vi "pumpsec_09_3.vi"(0 "reset":i32, 1 "master":i32, 2 "correction":dbl=1.0, 3 "manual":i32, 4 "pause":i32, 5 "Port":i32=10, 6 "pump_type":i32, 7 "port, Reglo D":i32, 10 "Target":dbl[](array[numeric])=[10.0, 2.0, 0.0, 0.0, 0.0, 0.0, 0.0, 0.0, 0.0, 0.0], 12 "fr_manual":dbl, 13 "Time":dbl[](array[numeric])=[4.0, 2.0, 0.0, 0.0, 0.0, 0.0, 0.0, 0.0, 0.0, 0.0]) -> (11 "Reglo D":dbl, 14 "Scale":dbl, 15 "mA":dbl format="%#_2g", 17 "Scale actual":dbl, 18 "params":dbl[](array[numeric]), 19 "PAM":dbl)   [LabVIEW 2015]
uses:
  BERTTA.dll
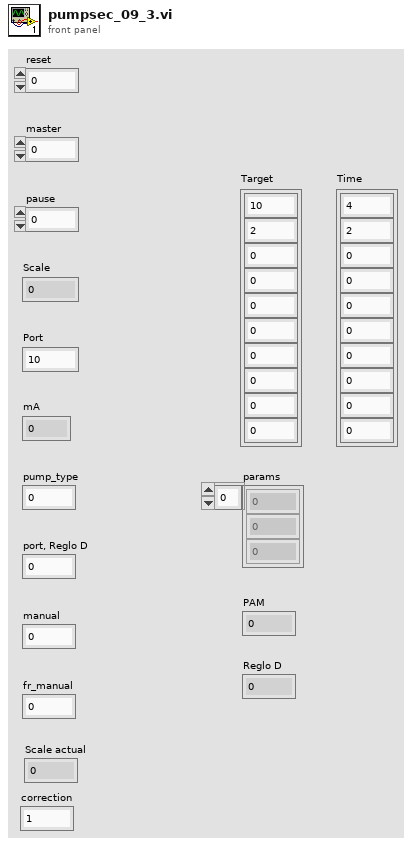
[diagram p1: front panel]
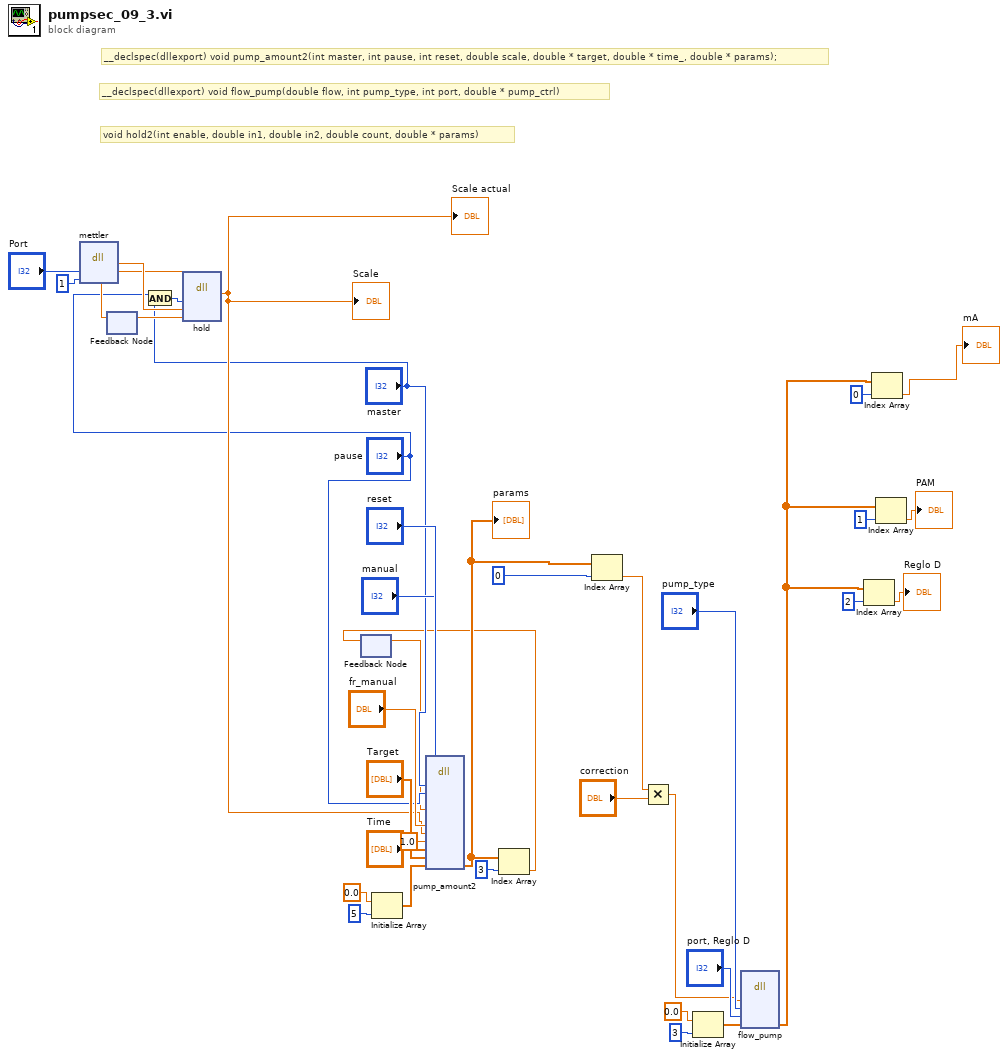
[diagram p0: block diagram]
diagram:
  # "void hold2(int enable, double in1, double in2, double count, double * params)"
  # "__declspec(dllexport) void flow_pump(double flow, int pump_type, int port, double * pump_ctrl)"
  # "__declspec(dllexport) void pump_amount2(int master, int pause, int reset, double scale, double * target, double * time_, double * params);"
  n1 = dll-call lib="C:/Users/shresplab/OneDrive - Kemira Oyj/Documents/Visual Studio 2017/Projects/Bertta/BERTTA/x64/Debug/BERTTA.dll" fn="mettler"("port"="Port", "msg"=1) -> ("return type"=w14:dbl)  [unwired: 5 in, 2 out]
  n2 = feedback #1() -> (w13:dbl)  [unwired: 1 in]
  n3 = And(x="pause", y="master") -> (x .and. y?=w9:i32)
  n4 = dll-call lib="C:/Users/shresplab/OneDrive - Kemira Oyj/Documents/Visual Studio 2017/Projects/Bertta/BERTTA/x64/Debug/BERTTA.dll" fn="hold"("enable"=w9, "in1"=w14, "in2"=w13) -> ("return type"=w12:dbl)  [unwired: 6 in, 2 out]
  "Scale" <- w12
  "Scale actual" <- w12
  n5 = feedback-in #1(w12) -> ()
  n6 = feedback #2() -> (w5:dbl)  [unwired: 1 in]
  n7 = Initialize Array(0.0 ("element"), 5 ("dimension size")) -> (w22:dbl[])
  n8 = dll-call lib="C:/Users/shresplab/OneDrive - Kemira Oyj/Documents/Visual Studio 2017/Projects/Bertta/BERTTA/x64/Debug/BERTTA.dll" fn="pump_amount2"("master"="master", "pause"="pause", "reset"="reset", "count"=w5, "manual"="manual", "fr_manual"="fr_manual", "scale"=w12, "elapsed"=1.0, "target"="Target", "time_"="Time", "params"=w22) -> ("params"=w7:dbl[])  [unwired: 14 in, 2 out]
  "params" <- w7
  n9 = Index Array(array=w7, index=3) -> (element=w6:dbl)
  n10 = feedback-in #2(w6) -> ()
  n11 = Index Array(array=w7, index=0) -> (element=w4:dbl)
  n12 = Multiply(x=w4, y="correction") -> (x*y=w3:dbl)
  n13 = Initialize Array(0.0 ("element"), 3 ("dimension size")) -> (w27:dbl[])
  n14 = dll-call lib="C:/Users/shresplab/OneDrive - Kemira Oyj/Documents/Visual Studio 2017/Projects/Bertta/BERTTA/x64/Debug/BERTTA.dll" fn="flow_pump"("flow"=w3, "pump_type"="pump_type", "port"="port, Reglo D", "pump_ctrl"=w27) -> ("pump_ctrl"=w18:dbl[])  [unwired: 7 in, 2 out]
  n15 = Index Array(array=w18, index=2) -> (element=→"Reglo D":dbl)
  n16 = Index Array(array=w18, index=0) -> (element=→"mA":dbl)
  n17 = Index Array(array=w18, index=1) -> (element=→"PAM":dbl)
